vi "Make circle of points.vi"(1 "Periphery":cluster{i32, i32}, 2 "Center":cluster{i32, i32}) -> (0 "Array of Points":cluster{"X":i32, "Y":i32}[](array[cluster]))   [LabVIEW 2011]
panel:
  in  "Number of points":i32=360
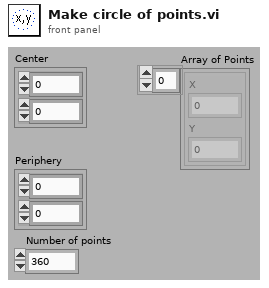
[diagram p1: front panel]
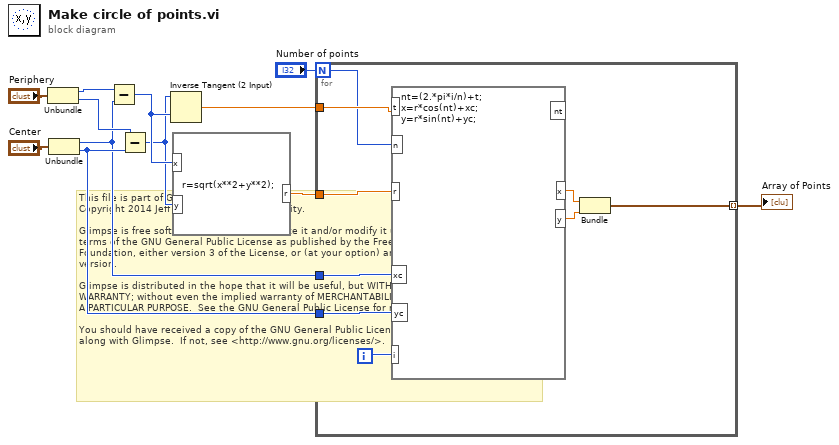
[diagram p0: block diagram]
diagram:
  # "This file is part of Glimpse. \nCopyright 2014 Jeff Gelles, Brandeis University.    \n\nGlimpse is free software: you can redistribute it and/or modify it under the \nterms of the GNU General Public License as published by the Free Software \nFoundation, either version 3 of the License, or (at your option) any later \nversion.\n\nGlimpse is distributed in the hope that it will be useful, but WITHOUT ANY \nWARRANTY; without even the implied warranty of MERCHANTABILITY or FITNESS FOR \nA PARTICULAR PURPOSE.  See the GNU General Public License for more details.\n\nYou should have received a copy of the GNU General Public License\nalong with Glimpse.  If not, see <http://www.gnu.org/licenses/>."
  n1 = Unbundle("Periphery") -> (w10:i32, w9:i32)
  n2 = Unbundle("Center") -> (w5:i32, w6:i32)
  n3 = Subtract(x=w10, y=w5) -> (x-y=w8:i32)
  n4 = Subtract(x=w9, y=w6) -> (x-y=w7:i32)
  n5 = Inverse Tangent (2 Input)(1:w8, 2:w7) -> (0:w3:dbl)
  n6 = formula code="r=sqrt(x**2+y**2);"("x"=w8, "y"=w7) -> ("r"=w4:dbl)
  n7 = for {
    N: "Number of points" -> [w16]
    tunnel: w6 -> [w20]
    tunnel: w5 -> [w19]
    tunnel: w4 -> [w18]
    tunnel: w3 -> [w17]
    tunnel: [w13] -> w1 mode=indexing
    i -> [w21]
    n8 = formula code="nt=(2.*pi*i/n)+t;\nx=r*cos(nt)+xc;\ny=r*sin(nt)+yc;"("r"=w18, "t"=w17, "xc"=w19, "yc"=w20, "i"=w21, "n"=w16) -> ("x"=w15:dbl, "y"=w14:dbl)  [unwired: 1 out]
    n9 = Bundle("x"=w15, "y"=w14) -> (w13:cluster{"x":dbl, "y":dbl})  [unwired: 1 out]
  }
  "Array of Points" <- w1
